vi "PPT_Check_reply.vi"(0 "Address":string, 1 "PPT reply":string) -> (3 "Stripped string":string, 4 "Error Notes":string)   [LabVIEW 2010]
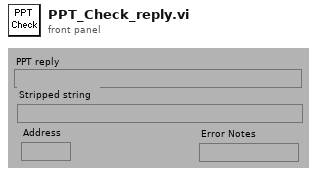
[diagram p1: front panel]
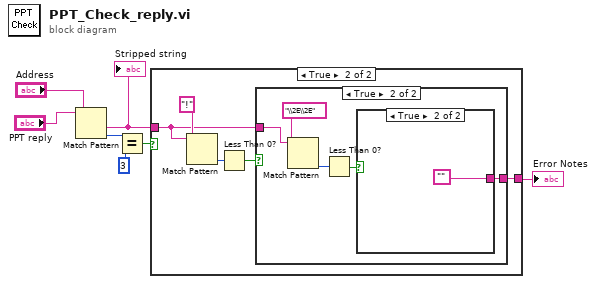
[diagram p0: block diagram]
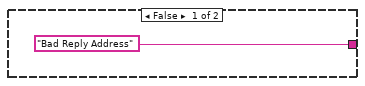
[diagram p2: hidden frame]
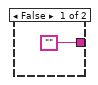
[diagram p3: hidden frame]
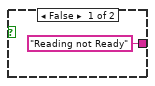
[diagram p4: hidden frame]
diagram:
  n1 = Match Pattern(string="PPT reply", regular expression="Address") -> (after substring=w1:string, offset past match=w5:i32)  [unwired: 3 out]
  "Stripped string" <- w1
  n2 = Equal?(x=w5, y=3) -> (x = y?=w3:bool)
  n3 = case shown="True" w3 {
    tunnel: ["Bad Reply Address" w10] -> w2
    tunnel: w1 -> [_ w9]
    frame False {
    }
    frame True {
      n4 = Match Pattern(string=w9, regular expression="!") -> (offset past match=w11:i32)  [unwired: 4 out]
      n5 = Less Than 0?(x=w11) -> (x < 0?=w12:bool)
      n6 = case shown="True" w12 {
        tunnel: ["" w15] -> w10
        tunnel: w9 -> [_ w18]
        frame False {
        }
        frame True {
          n7 = Match Pattern(string=w18, regular expression="\\2E\\2E") -> (offset past match=w17:i32)  [unwired: 4 out]
          n8 = Less Than 0?(x=w17) -> (x < 0?=w16:bool)
          n9 = case shown="True" w16 {
            tunnel: ["Reading not Ready" ""] -> w15
            frame False {
            }
            frame True {
            }
          }
        }
      }
    }
  }
  "Error Notes" <- w2
